vi "Debug Settings from ini.vi"(7 "Section":string, 8 "error in (no error)":errorcluster, 11 "Acquisition Settings In":T1) -> (0 "error out":errorcluster, 3 "Debug Settings Cluster":T1, 5 "All Tags Exists?":bool)   [LabVIEW 2013]
doc: "Loads the TCP port being used for listening for incoming connections."
uses:
  Debug/Debug Settings Cluster.ctl
  Debug Setting Enum Keys.ctl
  Common/File IO/INI/Read write mode.ctl
  Common/File IO/INI/INI Read write bool.vi
  Common/File IO/INI/INI Read write path.vi
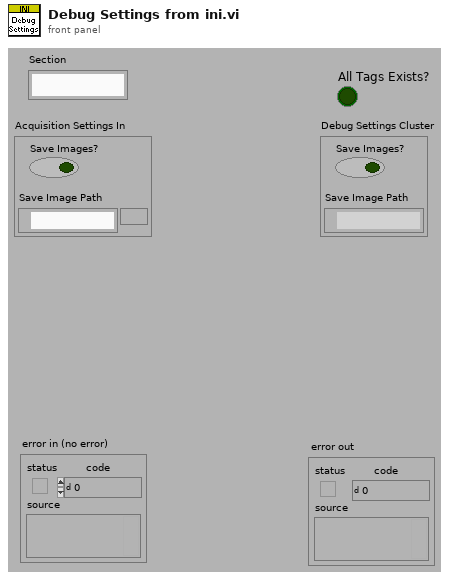
[diagram p1: front panel]
types:
  T1 = typedef "Debug Settings Cluster.ctl" = cluster{"Save Images?":bool, "Save Image Path":path}
  T2 = typedef "Debug Setting Enum Keys.ctl" = enum16{"Save Image", "Save Image Path"}
  T3 = typedef "Read write mode.ctl" = enum16{"Read", "Write"}
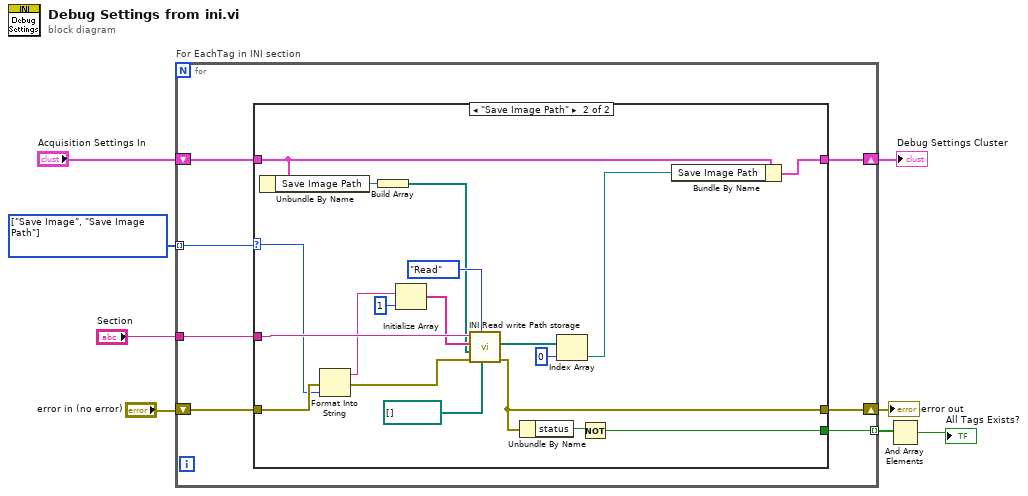
[diagram p0: block diagram]
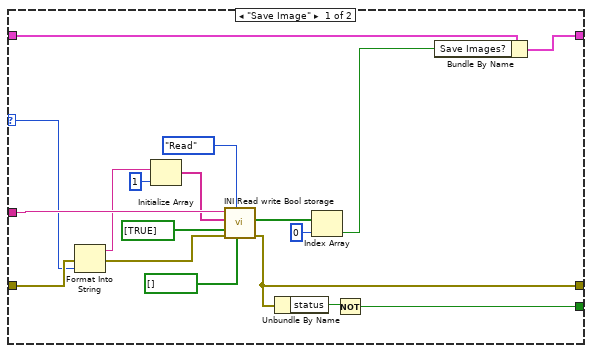
[diagram p2: hidden frame]
diagram:
  w8 = T2[] [enum."Save Image", enum."Save Image Path"] items=["Save Image", "Save Image Path"]
  n1 = for "For EachTag in INI section" {
    tunnel: "Section" -> [w15]
    tunnel: w8 -> [w14] mode=indexing
    shift-right: [w10] -> w6
    shift-left: "error in (no error)" -> [w12]
    shift-right: [w9] -> w1
    shift-left: "Acquisition Settings In" -> [w13]
    tunnel: [w11] -> w4 mode=indexing
    n2 = case shown="\"Save Image Path\"" w14 {
      selector: w14 -> [w28 w48]
      tunnel: w15 -> [w32 w51]
      tunnel: w13 -> [w30 w36]
      tunnel: w12 -> [w29 w49]
      tunnel: [w33 w52] -> w10
      tunnel: [w18 w38] -> w11
      tunnel: [w31 w50] -> w9
      frame "Save Image" {
        n3 = Format Into String(error in=w29, w28) -> (resulting string=w26:string, error out=w19:errorcluster)  [unwired: 2 in]
        n4 = Initialize Array(w26, 1 ("dimension size")) -> (w24:string[])
        n5 = call "INI Read write Bool storage.vi"("Values to write"=bool[] [], "Read/Write mode"=Read_write_mode."Read", "error in"=w19, "Defaults"=bool[] [TRUE], "keys"=w24, "section"=w32) -> ("error out"=w33:errorcluster, "Values"=w23:bool[])  [unwired: 4 in]
        n6 = Unbundle By Name(w33) -> ("status"=w20:bool)
        n7 = Index Array(array=w23, index=0) -> (element=w21:bool)
        n8 = Not(x=w20) -> (.not. x?=w18:bool)
        n9 = Bundle By Name(cluster=w30, "Save Images?"=w21) -> (w31:T1)
      }
      frame "Save Image Path" {
        n10 = Unbundle By Name(w36) -> ("Save Image Path"=w35:path)
        n11 = Format Into String(error in=w49, w48) -> (resulting string=w46:string, error out=w39:errorcluster)  [unwired: 2 in]
        n12 = Build Array(w35) -> (w34:path[])
        n13 = Initialize Array(w46, 1 ("dimension size")) -> (w44:string[])
        n14 = call "INI Read write Path storage.vi"("Values to write"=path[] [], "Read/Write mode"=Read_write_mode."Read", "error in"=w39, "Defaults"=w34, "keys"=w44, "section"=w51) -> ("error out"=w52:errorcluster, "Values"=w43:path[])  [unwired: 4 in]
        n15 = Unbundle By Name(w52) -> ("status"=w40:bool)
        n16 = Index Array(array=w43, index=0) -> (element=w41:path)
        n17 = Not(x=w40) -> (.not. x?=w38:bool)
        n18 = Bundle By Name(cluster=w36, "Save Image Path"=w41) -> (w50:T1)
      }
    }
  }
  "error out" <- w6
  "Debug Settings Cluster" <- w1
  n19 = And Array Elements(Boolean array=w4) -> (logical AND=→"All Tags Exists?":bool)
